vi "relative_time_to_string.vi"(1 "Seconds":ext) -> (0 "String time":string="0 days, 0 h, 0 m, 0 s.")   [LabVIEW 2013]
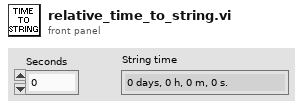
[diagram p1: front panel]
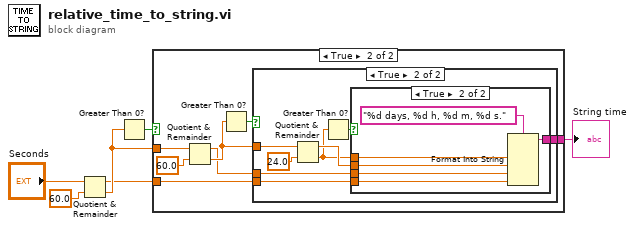
[diagram p0: block diagram]
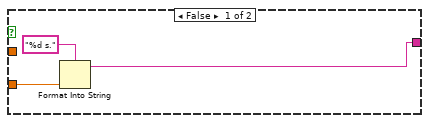
[diagram p2: hidden frame]
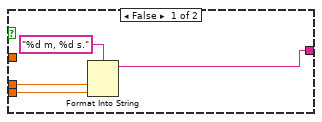
[diagram p3: hidden frame]
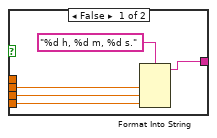
[diagram p4: hidden frame]
diagram:
  n1 = Quotient & Remainder(x="Seconds", y=60.0) -> (x-y*floor(x/y)=w2:ext, floor(x/y)=w4:ext)
  n2 = Greater Than 0?(x=w4) -> (x > 0?=w3:bool)
  n3 = case shown="True" w3 {
    tunnel: w4 -> [_ w15]
    tunnel: w2 -> [w8 w13]
    tunnel: [w7 w10] -> w1
    frame False {
      n4 = Format Into String(format string="%d s.", w8) -> (resulting string=w7:string)  [unwired: 2 in, 1 out]
    }
    frame True {
      n5 = Quotient & Remainder(x=w15, y=60.0) -> (x-y*floor(x/y)=w11:ext, floor(x/y)=w12:ext)
      n6 = Greater Than 0?(x=w12) -> (x > 0?=w14:bool)
      n7 = case shown="True" w14 {
        tunnel: w12 -> [_ w28]
        tunnel: w13 -> [w18 w25]
        tunnel: w11 -> [w19 w24]
        tunnel: [w17 w21] -> w10
        frame False {
          n8 = Format Into String(format string="%d m, %d s.", w19, w18) -> (resulting string=w17:string)  [unwired: 2 in, 1 out]
        }
        frame True {
          n9 = Quotient & Remainder(x=w28, y=24.0) -> (x-y*floor(x/y)=w23:ext, floor(x/y)=w22:ext)
          n10 = Greater Than 0?(x=w22) -> (x > 0?=w26:bool)
          n11 = case shown="True" w26 {
            tunnel: w25 -> [w32 w38]
            tunnel: w24 -> [w31 w37]
            tunnel: w23 -> [w30 w36]
            tunnel: w22 -> [_ w35]
            tunnel: [w29 w34] -> w21
            frame False {
              n12 = Format Into String(format string="%d h, %d m, %d s.", w30, w31, w32) -> (resulting string=w29:string)  [unwired: 2 in, 1 out]
            }
            frame True {
              n13 = Format Into String(format string="%d days, %d h, %d m, %d s.", w35, w36, w37, w38) -> (resulting string=w34:string)  [unwired: 2 in, 1 out]
            }
          }
        }
      }
    }
  }
  "String time" <- w1
